vi "ClearBuffer.vi"(8 "error in (no error)":errorcluster caption="错误输入（无错误）", 11 "ZLGCAN 输入":refnum<class "ZLGCAN.lvclass">) -> (0 "error out":errorcluster caption="错误输出", 3 "ZLGCAN 输出":refnum<class "ZLGCAN.lvclass">)   [LabVIEW 2020, in "ZLGCAN.lvclass"]
uses:
  ZLGCAN.lvclass
  ZLGCAN.lvclass/ZLGCAN.ctl
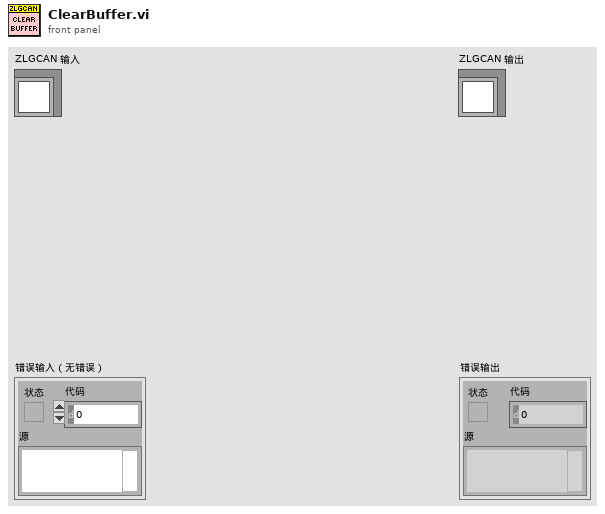
[diagram p1: front panel]
types:
  T1 = cluster{"Device Type":u32, "Device Index":u32, "CANInd":u32, "Baud(E_U)":u32}
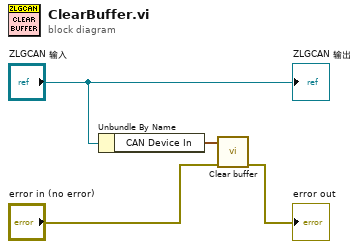
[diagram p0: block diagram]
diagram:
  n1 = Unbundle By Name("ZLGCAN 输入") -> ("CAN Device In"=w3:T1)
  n2 = call "Clear buffer.vi"("错误输入（无错误）"="error in (no error)", "CAN Device In"=w3) -> ("错误输出"=→"error out":errorcluster)  [unwired: 8 in, 1 out]
  "ZLGCAN 输出" <- "ZLGCAN 输入"
